vi "Untitled 3.vi"   [LabVIEW 2015]
uses:
  <vilib>/drjdpowell/SQLite Library/SQLite.lvlib
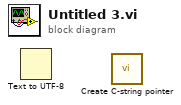
[diagram p0: block diagram]
diagram:
  n1 = Text to UTF-8() -> ()  [unwired: 3 in, 2 out]
  n2 = call <vilib>:"Create C-string pointer.vi"() -> ()  [unwired: 8 in, 4 out]
